vi "SubVI_Edge #.vi"(0 "Image in":T6, 5 "Parameter_Edge":T3={"ROI Descriptor"={"Global Rectangle"=[], "Contours"=[]}, "Edge Options"={"Edge Options"={"Edge Polarity"=0, "Kernel Size"=3, "Width"=3, "Minimum Edge Strength"=10.0, "Interpolation Type"=enum."Bilinear Fixed", "Data Processing Method"=enum."Average"}, "Scan Direction"=0, "Step Size"=5, "SD"=0.0, "Auto"=FALSE}, "條件(Line)"={"毛邊長度"=5.0}} {"ROI Descriptor"."Contours"."Type" items=["No Selection", "Point", "Line", "Rectangle", "Oval", "Polygon", "Free", "Annulus", "Unused2", "Unused3", "Broken Line", "Free Hand Line", "Rotated Rectangle"]; "Edge Options"."Edge Options"."Edge Polarity" items=["All Edges", "Rising Edges", "Falling Edges"]; "Edge Options"."Edge Options"."Minimum Edge Strength" format="%.2f"; "Edge Options"."Edge Options"."Width" step=2; "Edge Options"."Edge Options"."Kernel Size" step=2; "Edge Options"."Scan Direction" items=["Left To Right", "Right To Left", "Top To Bottom", "Bottom To Top"]}, 11 "error in":errorcluster) -> (4 "Image Out":T6, 6 "Perpendicular Line":T2, 8 "Fit Line":T1, 10 "Distance":dbl, 15 "error out":errorcluster)   [LabVIEW 2013]
uses:
  <vilib>/vision/Image Controls.llb/IMAQ Image.ctl
  Control/Control Find Edge #.ctl
  <vilib>/vision/Measure.llb/Edge Options.ctl
  <vilib>/vision/Measure.llb/Edge Polarity.ctl
  <vilib>/vision/NI_Vision_Development_Module.lvlib
  <vilib>/Analysis/NI_AALBase.lvlib
  <vilib>/Analysis/NI_AALPro.lvlib
  <vilib>/Analysis/6fits.llb/Curve Fitting Criteria.ctl
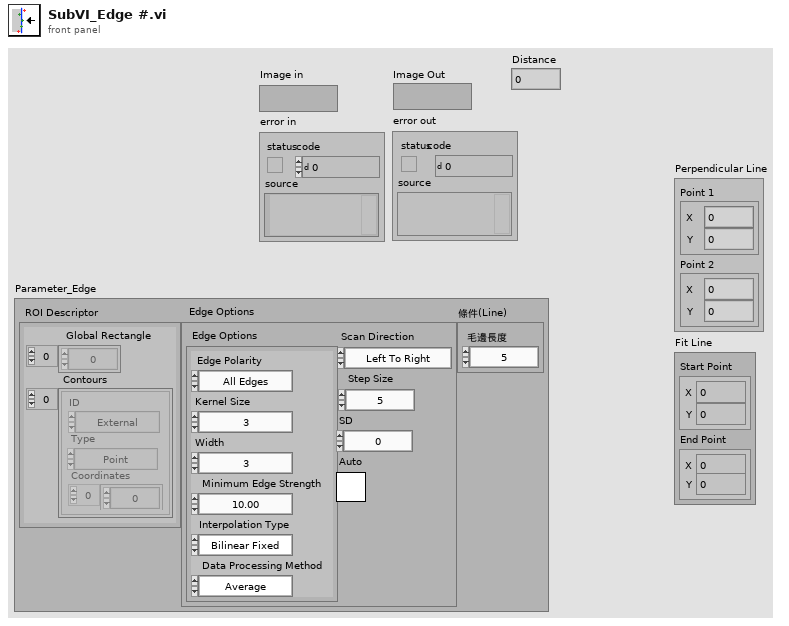
[diagram p1: front panel]
types:
  T1 = cluster{"Start Point":cluster{"X":i32, "Y":i32}, "End Point":cluster{"X":i32, "Y":i32}}
  T2 = cluster{"Point 1":cluster{"X":i32, "Y":i32}, "Point 2":cluster{"X":i32, "Y":i32}}
  T3 = typedef "Control Find Edge #.ctl" = cluster{"ROI Descriptor":cluster{"Global Rectangle":i32[], "Contours":cluster{"ID":enum32{"External", "Internal"}, "Type":u32, "Coordinates":i32[]}[]}, "Edge Options":cluster{"Edge Options":T4, "Scan Direction":u16, "Step Size":u32, "SD":dbl, "Auto":bool}, "條件(Line)":cluster{"毛邊長度":dbl}}
  T4 = typedef "Edge Options.ctl" = cluster{"Edge Polarity":T5, "Kernel Size":u32, "Width":u32, "Minimum Edge Strength":sgl, "Interpolation Type":enum32{"Zero Order", "Bilinear", "Quadratic", "Cubic", "Bilinear Fixed"}, "Data Processing Method":enum32{"Average", "Median"}}
  T5 = typedef "Edge Polarity.ctl" = u32
  T6 = typedef "IMAQ Image.ctl" = refnum<image>
  T7 = cluster{"Global Rectangle":i32[], "Contours":cluster{"ID":enum32{"External", "Internal"}, "Type":u32, "Coordinates":i32[]}[]}
  T8 = cluster{"Edge Options":T4, "Scan Direction":u16, "Step Size":u32, "SD":dbl, "Auto":bool}
  T9 = typedef "NI_AALPro.lvlib/Curve Fitting Criteria.ctl" = u16
  T10 = cluster{cluster{"X":dbl, "Numeric":dbl}, cluster{"X":dbl, "Numeric":dbl}}
  T11 = cluster{"Point 1":cluster{"X":sgl, "Y":sgl}, "Point 2":cluster{"X":sgl, "Y":sgl}}
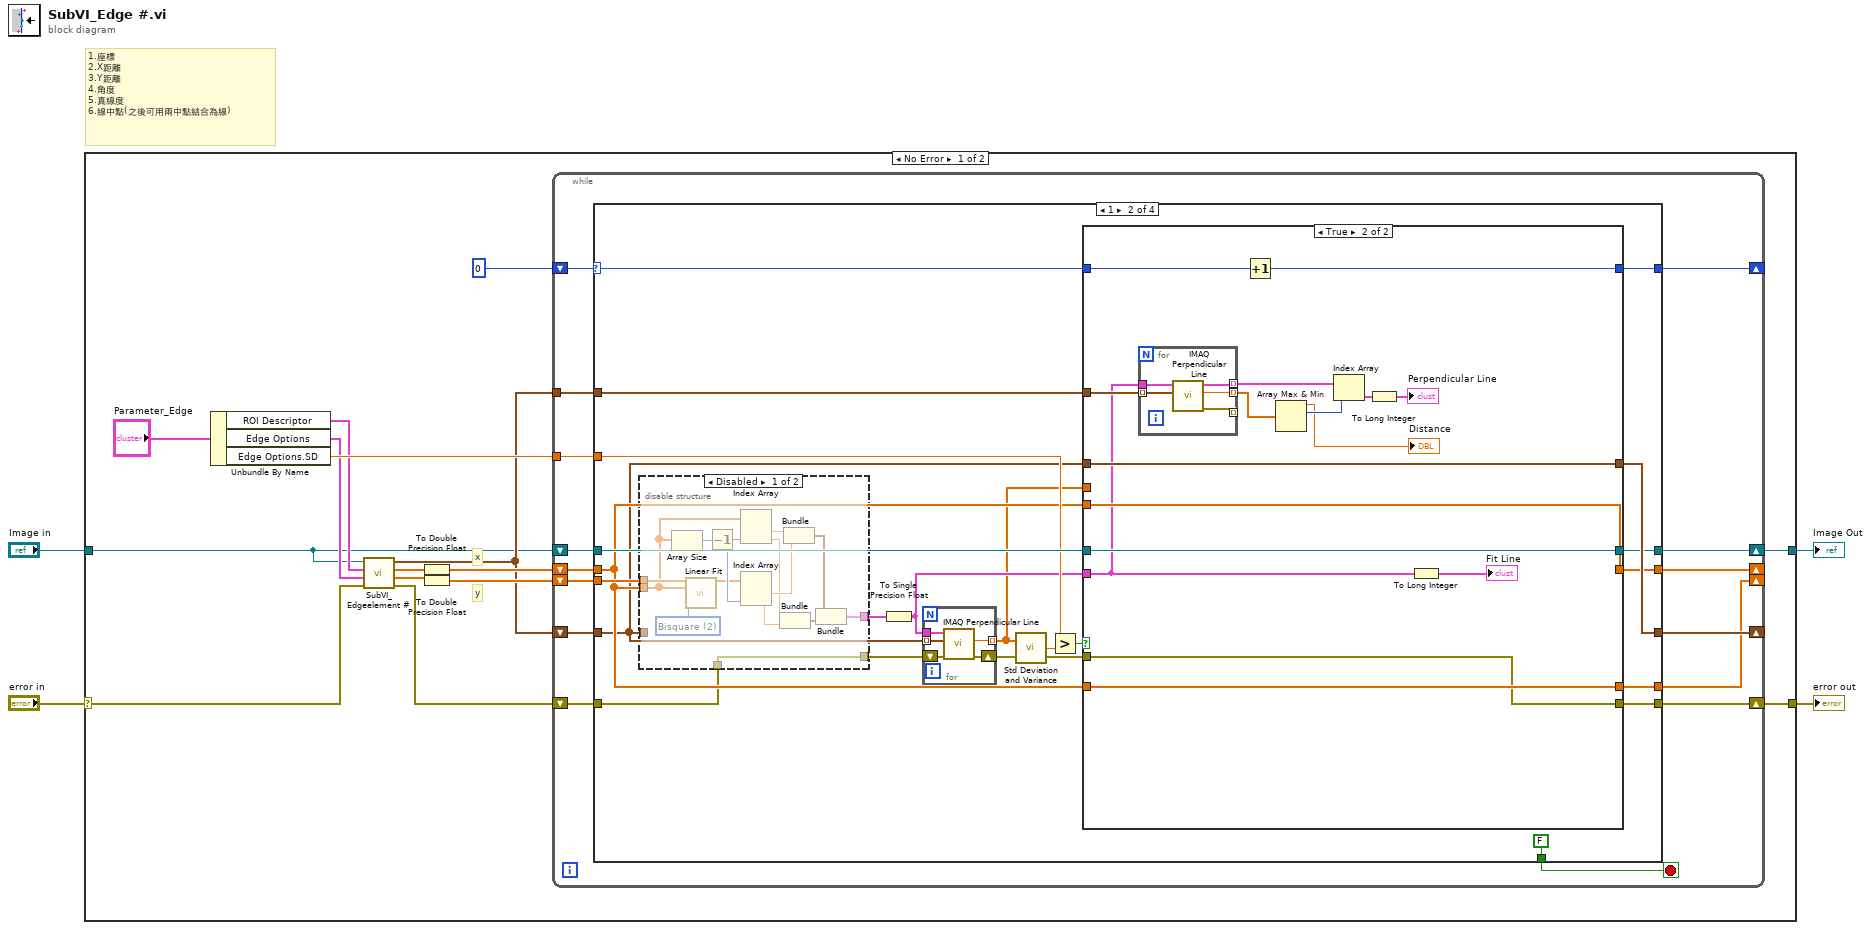
[diagram p0: block diagram]
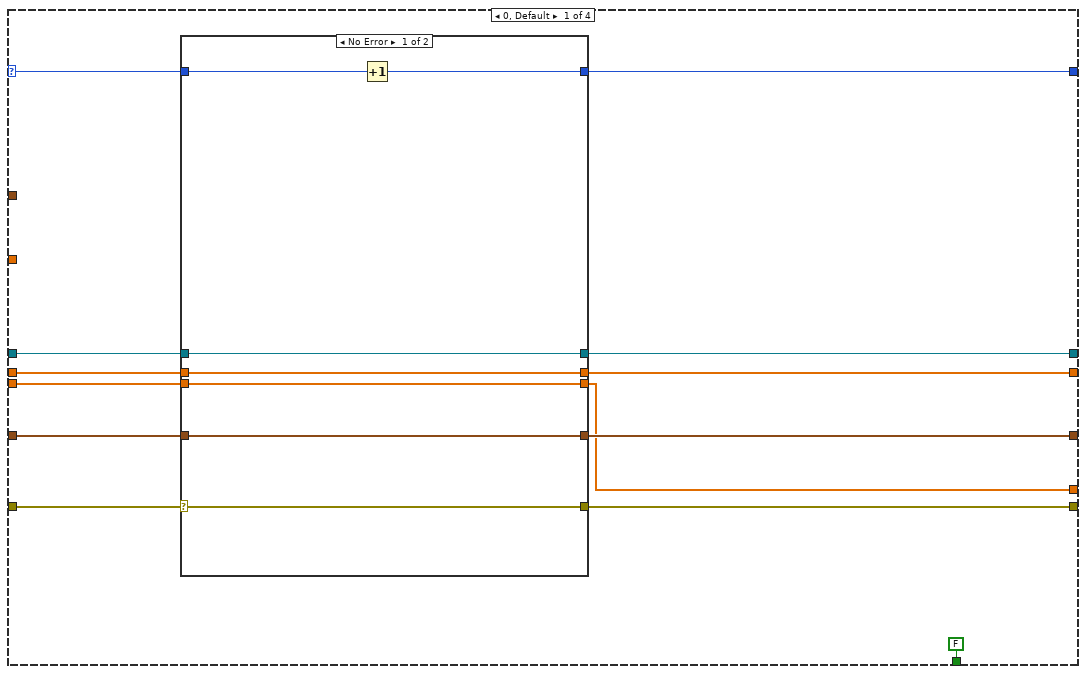
[diagram p2: hidden frame]
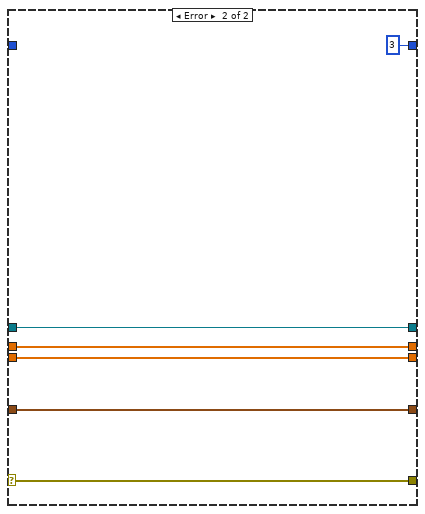
[diagram p3: hidden frame]
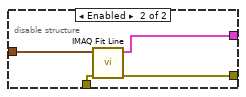
[diagram p4: hidden frame]
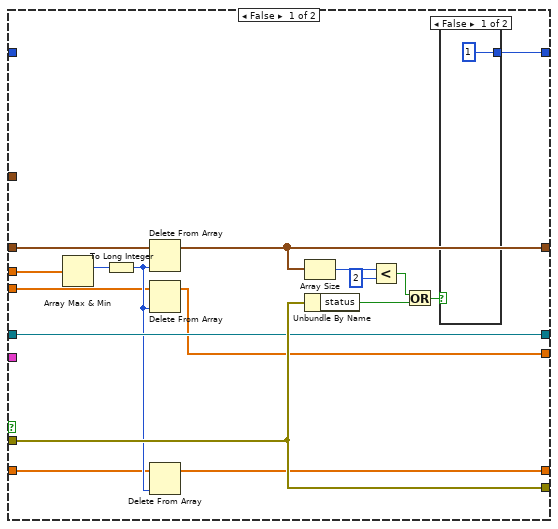
[diagram p5: hidden frame]
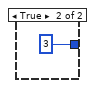
[diagram p6: hidden frame]
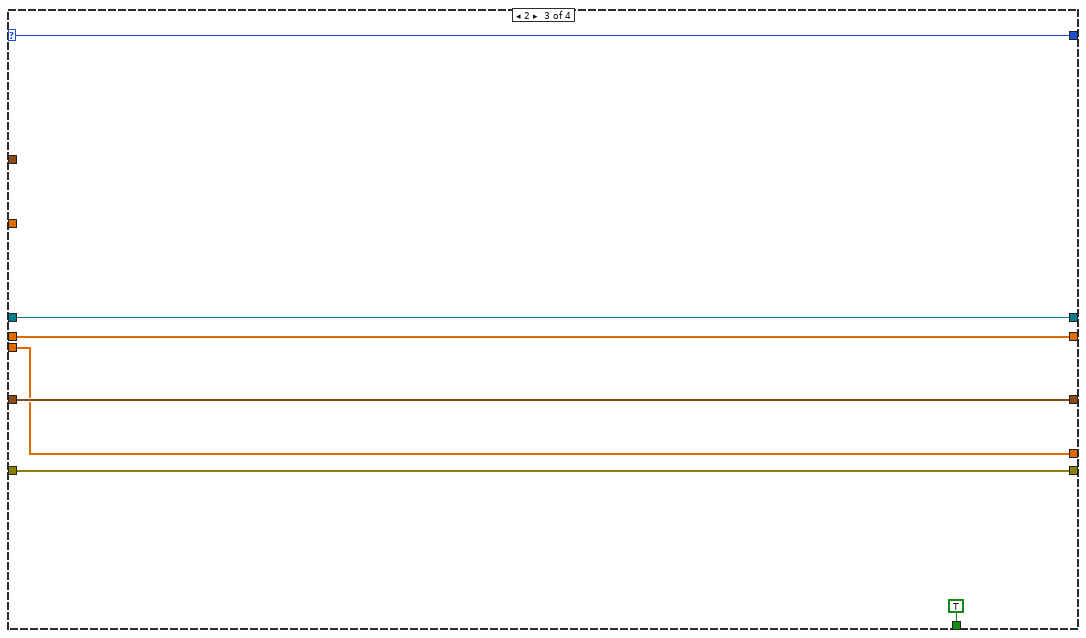
[diagram p7: hidden frame]
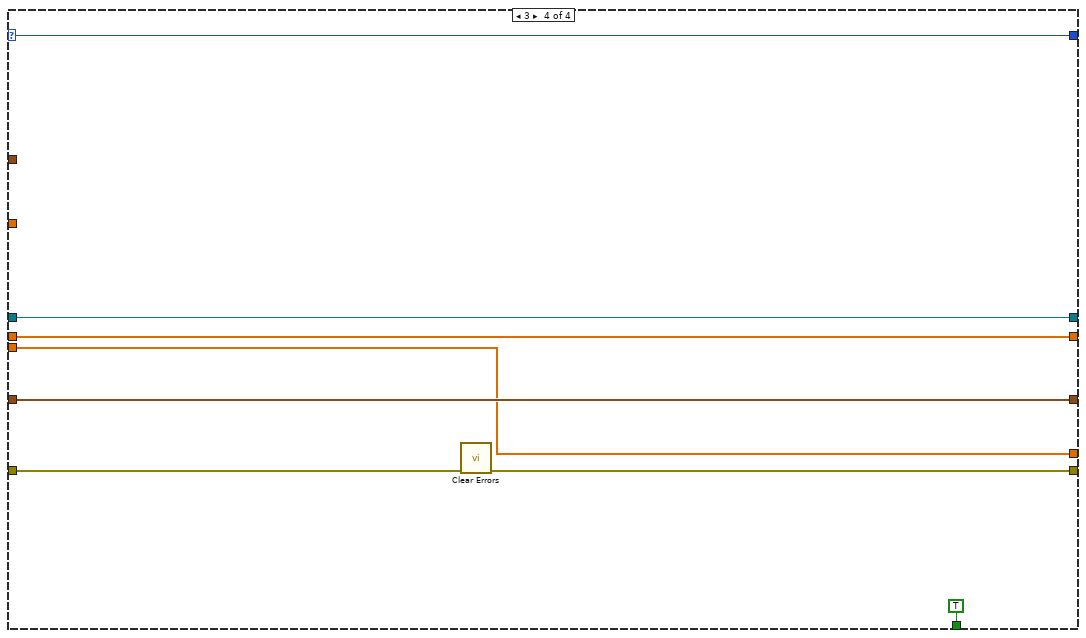
[diagram p8: hidden frame]
diagram:
  # "1.座標\n2.X距離\n3.Y距離\n4.角度\n5.真線度\n6.線中點(之後可用兩中點結合為線)"
  n1 = case shown="No Error" "error in" {
    selector: "error in" -> [w17 w162]
    tunnel: "Image in" -> [w5 w161]
    tunnel: [w16 w162] -> w2
    tunnel: [w15 w161] -> w1
    frame No Error {
      # "y"
      # "x"
      n2 = Unbundle By Name("Parameter_Edge") -> ("ROI Descriptor"=w8:T7, "Edge Options"=w7:T8, "Edge Options.SD"=w9:dbl)
      n3 = call "SubVI_Edgeelement #.vi"("Error In"=w17, "Parameter_Edge"=w7, "ROI Descriptor"=w8, "Image In"=w5) -> ("Error Out"=w18:errorcluster, "Y Array"=w10:sgl[], "X Array"=w11:sgl[], "Location"=w6:cluster{"X":sgl, "Y":sgl}[])  [unwired: 4 in]
      n4 = To Double Precision Float(number=w11) -> (double precision float=w14:dbl[])
      n5 = To Double Precision Float(number=w10) -> (double precision float=w13:dbl[])
      n6 = while {
        shift-right: [w32] -> _
        shift-left: 0 -> [w34]
        shift-right: [w31] -> w16
        shift-left: w18 -> [w33]
        shift-right: [w29] -> _
        shift-left: w6 -> [w30]
        shift-right: [w27] -> w15
        shift-left: w5 -> [w28]
        tunnel: w9 -> [w25]
        shift-right: [w22] -> _
        shift-left: w14 -> [w24]
        shift-right: [w21] -> _
        shift-left: w13 -> [w23]
        tunnel: w6 -> [w20]
        stop <- w26 stop-if-true
        n7 = case shown="1" w34 {
          selector: w34 -> [w43 w74 w149 w155]
          tunnel: w33 -> [w41 w62 w152 w160]
          tunnel: [w42 w75 w149 w155] -> w32
          tunnel: [w45 w76 w152 w159] -> w31
          tunnel: [w39 w80 w150 w157] -> w29
          tunnel: w30 -> [w40 w63 w150 w157]
          tunnel: w28 -> [w47 w79 w151 w158]
          tunnel: [w46 w78 w151 w158] -> w27
          tunnel: [FALSE FALSE TRUE TRUE] -> w26
          tunnel: w25 -> [_ w72 _ _]
          tunnel: w24 -> [w38 w70 w147 w154]
          tunnel: w23 -> [w36 w71 w146 w153]
          tunnel: [w37 w69 w147 w154] -> w22
          tunnel: [w35 w68 w146 w153] -> w21
          tunnel: w20 -> [_ w65 _ _]
          frame 0, Default {
            n8 = case shown="No Error" w41 {
              selector: w41 -> [w51 w58]
              tunnel: w47 -> [w50 w59]
              tunnel: [w50 w59] -> w46
              tunnel: [w51 w58] -> w45
              tunnel: w43 -> [w54 _]
              tunnel: [w53 3] -> w42
              tunnel: w40 -> [w52 w57]
              tunnel: [w52 w57] -> w39
              tunnel: w38 -> [w49 w56]
              tunnel: [w49 w56] -> w37
              tunnel: w36 -> [w48 w55]
              tunnel: [w48 w55] -> w35
              frame No Error {
                n9 = Increment(x=w54) -> (x+1=w53:i32)
              }
              frame Error {
              }
            }
          }
          frame 1 {
            n10 = disable-structure shown="Disabled" {
              disable-tunnel: w71 -> [w95 _]
              disable-tunnel: w70 -> [w87 _]
              disable-tunnel: [w86 w99] -> w67
              disable-tunnel: w63 -> [_ w100]
              disable-tunnel: w62 -> [w83 w98]
              disable-tunnel: [w83 w97] -> w61
              frame Disabled {
                w84 = T9 2 items=["Least Square", "Least Absolute Residual", "Bisquare"] ("method")
                n11 = Array Size(array=w87) -> (size(s)=w96:i32)
                n12 = call <vilib>:"Linear Fit.vi"("Y"=w95, "X"=w87, "method"=w84) -> ("Best Linear Fit"=w85:dbl[])  [unwired: 8 in, 4 out]
                n13 = Decrement(x=w96) -> (x-1=w88:i32)
                n14 = Index Array(array=w87, index #2=w88) -> (element #1=w94:dbl, element #2=w92:dbl)  [unwired: 1 in]
                n15 = Index Array(array=w85, index #2=w88) -> (element #1=w93:dbl, element #2=w91:dbl)  [unwired: 1 in]
                n16 = Bundle("X"=w92, "Numeric"=w91) -> (w89:cluster{"X":dbl, "Numeric":dbl})  [unwired: 1 in]
                n17 = Bundle("X"=w94, "Numeric"=w93) -> (w90:cluster{"X":dbl, "Numeric":dbl})  [unwired: 1 in]
                n18 = Bundle(w90, w89) -> (w86:T10)  [unwired: 1 in]
              }
              frame Enabled {
                n19 = call "IMAQ Fit Line"("error in (no error)"=w98, "Points"=w100) -> ("error out"=w97:errorcluster, "Line Segment"=w99:T11)  [unwired: 4 in, 4 out]
              }
            }
            n20 = To Single Precision Float(number=w67) -> (single precision float=w66:T11)
            n21 = for {
              tunnel: w66 -> [w145]
              tunnel: w63 -> [w144] mode=indexing
              tunnel: [w143] -> w64 mode=indexing
              shift-right: [w141] -> w77
              shift-left: w61 -> [w142]
              n22 = call "IMAQ Perpendicular Line"("error in (no error)"=w142, "Point"=w144, "Line"=w145) -> ("error out"=w141:errorcluster, "Distance"=w143:dbl)  [unwired: 6 in, 1 out]
            }
            n23 = call <vilib>:"Std Deviation and Variance.vi"("X"=w64) -> ("standard deviation"=w82:dbl)  [unwired: 1 in, 2 out]
            n24 = Greater?(x=w72, y=w82) -> (0:w81:bool)
            n25 = case shown="True" w81 {
              tunnel: w63 -> [w117 w133]
              tunnel: [w113 w133] -> w80
              tunnel: w79 -> [w107 w130]
              tunnel: [w107 w130] -> w78
              tunnel: w77 -> [w108 w129]
              tunnel: [w108 w129] -> w76
              tunnel: [w115 w134] -> w75
              tunnel: w74 -> [_ w135]
              tunnel: w66 -> [_ w122]
              tunnel: w70 -> [w105 w131]
              tunnel: w70 -> [w104 w132]
              tunnel: [w103 w131] -> w69
              tunnel: [w102 w132] -> w68
              tunnel: w65 -> [_ w128]
              tunnel: w64 -> [w101 _]
              frame False {
                n26 = Array Max & Min(array=w101) -> (max index (indices)=w116:i32)  [unwired: 3 out]
                n27 = To Long Integer(number=w116) -> (32bit integer=w106:i32)
                n28 = Delete From Array(array=w117, index=w106) -> (array with subset deleted=w113:cluster{"X":sgl, "Y":sgl}[])  [unwired: 1 in, 1 out]
                n29 = Delete From Array(array=w105, index=w106) -> (array with subset deleted=w103:dbl[])  [unwired: 1 in, 1 out]
                n30 = Delete From Array(array=w104, index=w106) -> (array with subset deleted=w102:dbl[])  [unwired: 1 in, 1 out]
                n31 = Array Size(array=w113) -> (size(s)=w112:i32)
                n32 = Unbundle By Name(w108) -> ("status"=w114:bool)
                n33 = Less?(x=w112, y=2) -> (x < y?=w110:bool)
                n34 = Or(x=w110, y=w114) -> (x .or. y?=w109:bool)
                n35 = case shown="False" w109 {
                  tunnel: [1 3] -> w115
                  frame False {
                  }
                  frame True {
                  }
                }
              }
              frame True {
                n36 = for {
                  tunnel: w128 -> [w140] mode=indexing
                  tunnel: w122 -> [w139]
                  tunnel: [w138] -> w127 mode=indexing
                  tunnel: [w137] -> w126 mode=indexing
                  tunnel: [w136] -> _ mode=indexing
                  n37 = call "IMAQ Perpendicular Line"("Point"=w140, "Line"=w139) -> ("error out"=w136:errorcluster, "Distance"=w138:dbl, "Perpendicular Line"=w137:T11)  [unwired: 7 in]
                }
                n38 = Increment(x=w135) -> (x+1=w134:i32)
                n39 = Array Max & Min(array=w127) -> (max value=→"Distance":dbl, max index (indices)=w125:i32)  [unwired: 2 out]
                n40 = Index Array(array=w126, index=w125) -> (element=w124:T11)
                n41 = To Long Integer(number=w124) -> (32bit integer=→"Perpendicular Line":T2)
                n42 = To Long Integer(number=w122) -> (32bit integer=→"Fit Line":T2)
              }
            }
          }
          frame 2 {
          }
          frame 3 {
            n43 = call <vilib>:"Clear Errors.vi"("error in (no error)"=w160) -> ("error out"=w159:errorcluster)  [unwired: 6 in]
          }
        }
      }
    }
    frame Error {
    }
  }
  "error out" <- w2
  "Image Out" <- w1
